vi "LOERN_GetImage.vi"(0 "XRef":T4, 1 "State In":T3={"Inputs"=1}) -> (14 "Image":T2, 15 "Fatal Error Out":T1)   [LabVIEW 2016, in "LV Object Event Registration Node.xnode"]
uses:
  LV Object Event Registration Node.xnode
  <vilib>/XNodeSupport/XNodeXNodeRef.ctl
  LOERN_State.ctl
  <vilib>/XNodeSupport/XNodeImage.ctl
  <vilib>/XNodeSupport/XNodeErrorCluster.ctl
  <vilib>/XNodeSupport/NI_XNodeSupport.lvlib
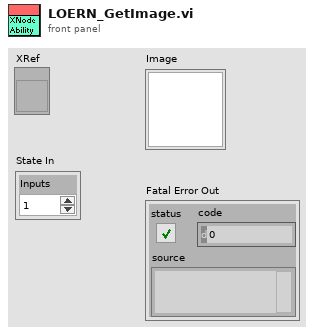
[diagram p1: front panel]
types:
  T1 = typedef "NI_XNodeSupport.lvlib/XNodeErrorCluster.ctl" = errorcluster
  T2 = typedef "NI_XNodeSupport.lvlib/XNodeImage.ctl" = picture
  T3 = typedef "LV Object Event Registration Node.xnode/LOERN_State.ctl" = cluster{"Inputs":u16}
  T4 = typedef "NI_XNodeSupport.lvlib/XNodeXNodeRef.ctl" = refnum<vi>
  T5 = cluster{"left":i16, "top":i16, "right":i16, "bottom":i16}
  T6 = cluster{"horizontal":enum16{"left", "center", "right"}, "vertical":enum16{"top", "center", "bottom"}}
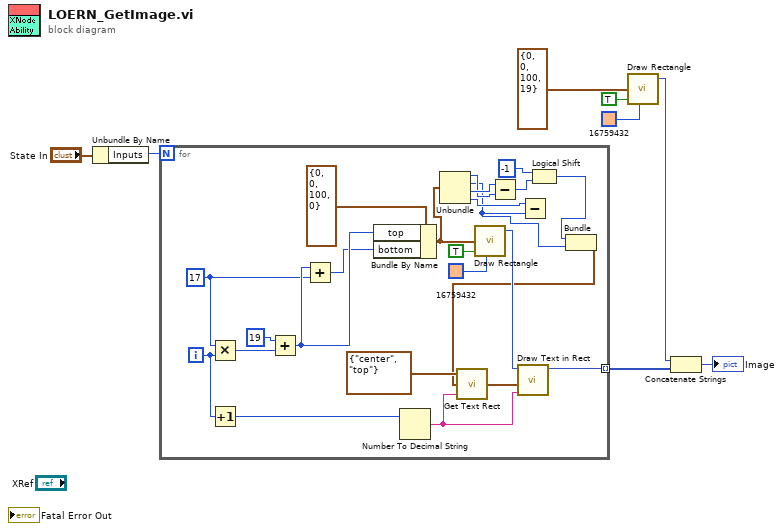
[diagram p0: block diagram]
diagram:
  n1 = Unbundle By Name("State In") -> ("Inputs"=w7:u16)
  n2 = for {
    N: w7 -> [_]
    tunnel: [w26] -> w1 mode=indexing
    i -> [w24]
    w19 = 17 ("x")
    n3 = Multiply(x=w19, y=w24) -> (x*y=w23:i32)
    n4 = Increment(x=w24) -> (x+1=w30:i32)
    n5 = Add(x=19, y=w23) -> (x+y=w20:i32)
    n6 = Add(x=w20, y=w19) -> (x+y=w18:i32)
    n7 = Bundle By Name(cluster=T5 {"left"=0, "top"=0, "right"=100, "bottom"=0} ("rect"), "top"=w20, "bottom"=w18) -> (w17:T5)
    n8 = Number To Decimal String(number=w30) -> (decimal integer string=w25:string)  [unwired: 1 in]
    n9 = Unbundle(w17) -> ("left"=w15:i16, "top"=w9:i16, "right"=w16:i16, "bottom"=w14:i16)
    n10 = call <vilib>:"Draw Rectangle.vi"("rect"=w17, "fill?(F)"=TRUE, "color(black)"=u32 16759432) -> ("new picture"=w27:picture)  [unwired: 6 in]
    n11 = Subtract(x=w16, y=w15) -> (x-y=w13:i16)
    n12 = Subtract(x=w14, y=w9) -> ()  [unwired: 1 out]
    n13 = Logical Shift(y=i16 -1, x=w13) -> (x << y=w11:i16)
    n14 = Bundle(w11, "top"=w9) -> (w10:cluster{i16, "top":i16})  [unwired: 1 in]
    n15 = call <vilib>:"Get Text Rect.vi"("alignment(left, top)"=T6 {"horizontal"=enum."center", "vertical"=enum."top"}, "origin(0,0)"=w10, "text"=w25) -> ("rect"=w31:T5)  [unwired: 6 in]
    n16 = call <vilib>:"Draw Text in Rect.vi"("text"=w25, "rect"=w31, "picture"=w27) -> ("new picture"=w26:picture)  [unwired: 8 in]
  }
  n17 = call <vilib>:"Draw Rectangle.vi"("rect"=T5 {"left"=0, "top"=0, "right"=100, "bottom"=19}, "fill?(F)"=TRUE, "color(black)"=u32 16759432) -> ("new picture"=w3:picture)  [unwired: 6 in]
  n18 = Concatenate Strings(w3, w1) -> (→"Image":picture)
